vi "Array-Dimensions (2D).vi"(7 "2D Array":dbl[][](array[numeric])) -> (6 "# rows":i32, 10 "# columns":i32)   [LabVIEW 2020]
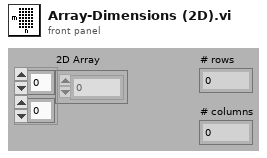
[diagram p1: front panel]
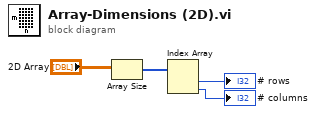
[diagram p0: block diagram]
diagram:
  n1 = Array Size(array="2D Array") -> (size(s)=w4:i32[])
  n2 = Index Array(array=w4) -> (element #1=→"# rows":i32, element #2=→"# columns":i32)  [unwired: 2 in]
